vi "Save Screenshot.vi"(8 "error in (no error)":errorcluster, 10 "Screen Shot Path":path, 11 "DPO4104 in":refnum<class "DPO4104.lvclass">) -> (0 "error out":errorcluster, 3 "DPO4104 out":refnum<class "DPO4104.lvclass">)   [LabVIEW 2018, in "DPO4104.lvlib" / "DPO4104.lvclass"]
doc: "This Override method is used to save a screen shot of the Oscope screen."
uses:
  DPO4104.lvclass
  PPLs/Oscilloscope/Parent/Oscilloscope.lvlibp/Oscilloscope.lvclass
  C:/Projects/LabVIEW/PPLs/Oscilloscope/Parent/Oscilloscope.lvlibp/Oscilloscope.lvclass
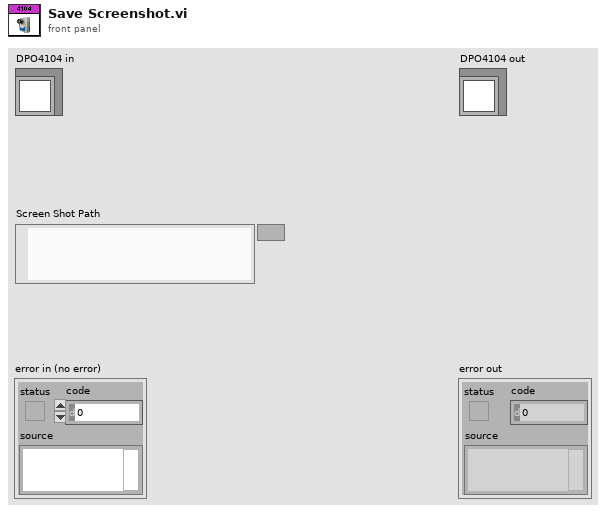
[diagram p1: front panel]
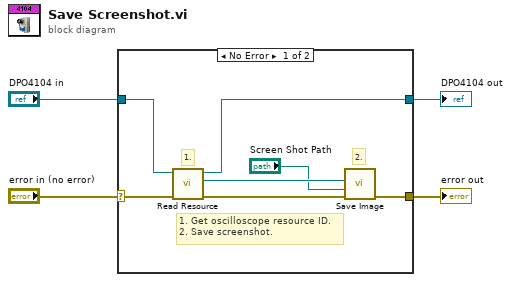
[diagram p0: block diagram]
diagram:
  n1 = case shown="No Error" "error in (no error)" {
    selector: "error in (no error)" -> [w11 w12]
    tunnel: [w6 w12] -> w3
    tunnel: [w9 w13] -> w1
    tunnel: "DPO4104 in" -> [w10 w13]
    frame No Error {
      # "2."
      # "1."
      # "1. Get oscilloscope resource ID.\n2. Save screenshot."
      n2 = call "Read Resource.vi"("error in (no error)"=w11, "Oscilloscope in"=w10) -> ("error out"=w7:errorcluster, "Resource"=w8:refnum<visa-resource-name>, "Oscilloscope out"=w9:refnum<class "DPO4104.lvclass">)  [unwired: 7 in]
      n3 = call "Save Image.vi"("error in (no error)"=w7, "Screen Shot Path"="Screen Shot Path", "VISA resource name"=w8) -> ("error out"=w6:errorcluster)  [unwired: 7 in, 1 out]
    }
    frame Error {
    }
  }
  "error out" <- w3
  "DPO4104 out" <- w1
